vi "State-Machine_Exercise1.vi"() -> ()   [LabVIEW 2019]
uses:
  State_Machine_states.ctl
panel:
  out "Measured Value Display":dbl
  in  "Measure Value":bool
  in  "Add to Chart":bool
  in  "Auto-Add Theashold":dbl(slide) scale=0.0..1.0
  out "Waveform Chart":dbl(graph)
  in  "stop":bool
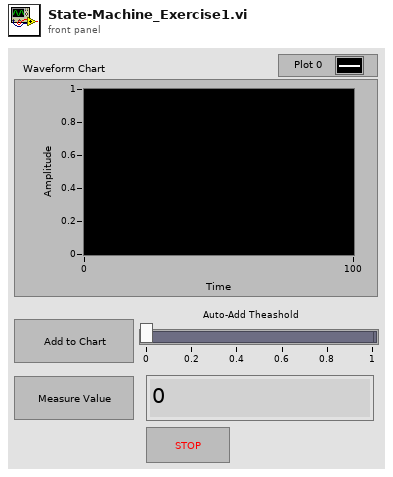
[diagram p1: front panel]
types:
  T1 = typedef "State_Machine_states.ctl" = enum16{"Idle", "Measure", "Display"}
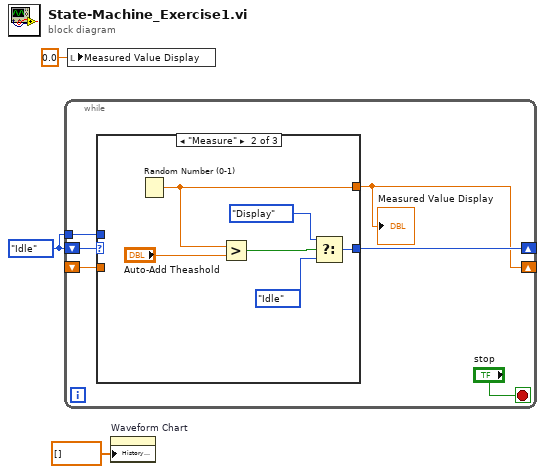
[diagram p0: block diagram]
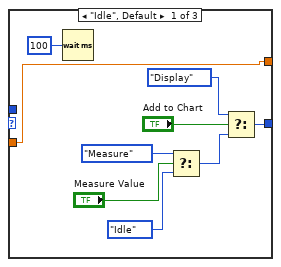
[diagram p2: hidden frame]
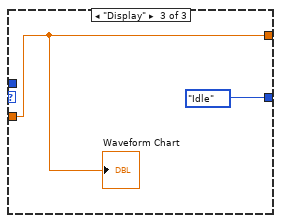
[diagram p3: hidden frame]
diagram:
  w3 = State_Machine_states."Idle"
  n1 = while {
    shift-right: [w8] -> _
    shift-left: w3 -> [w9]
    shift-right: [w5] -> _
    shift-left: _ -> [w6]
    tunnel: w3 -> [w4]
    stop <- "stop" stop-if-true
    n2 = case shown="\"Measure\"" w9 {
      tunnel: [w10 w24 State_Machine_states."Idle"] -> w8
      tunnel: w6 -> [w17 _ w26]
      tunnel: [w17 w20 w26] -> w5
      tunnel: w4 -> [_ _ _]
      frame "Idle", Default {
        n3 = Wait (ms)(milliseconds to wait=u32 100) -> ()  [unwired: 1 out]
        n4 = Select(t=State_Machine_states."Measure", s="Measure Value", f=State_Machine_states."Idle") -> (s? t:f=w13:T1)
        n5 = Select(t=State_Machine_states."Display", s="Add to Chart", f=w13) -> (s? t:f=w10:T1)
      }
      frame "Measure" {
        n6 = Random Number (0-1)() -> (number: 0 to 1=w20:dbl)
        n7 = Greater?(x=w20, y="Auto-Add Theashold") -> (0:w21:bool)
        n8 = Select(t=State_Machine_states."Display", s=w21, f=State_Machine_states."Idle") -> (s? t:f=w24:T1)
      }
      frame "Display" {
        "Waveform Chart" <- w26
      }
    }
    "Measured Value Display" <- w5
  }
  n9 = local write "Measured Value Display"(0.0 ("Measured Value Display")) -> ()
  n10 = property on="Waveform Chart" class="WFChart (strict)"("History Data"=dbl[] []) -> ()  [unwired: 2 in, 2 out]
